vi "题目 3.vi"() -> ()   [LabVIEW 2017]
panel:
  out "数组":dbl[][](array[numeric])
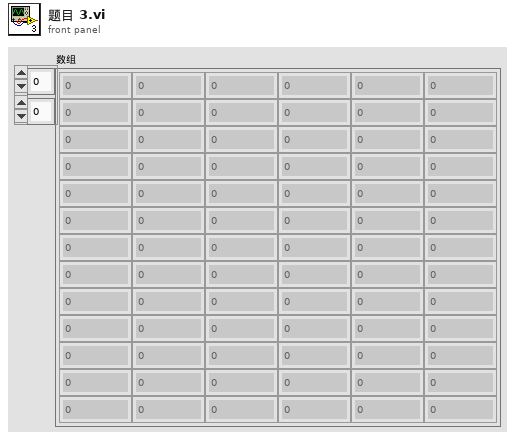
[diagram p1: front panel]
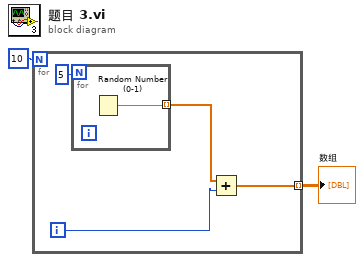
[diagram p0: block diagram]
diagram:
  n1 = for {
    N: 10 -> [_]
    tunnel: [w5] -> w1 mode=indexing
    i -> [w3]
    n2 = for {
      N: 5 -> [_]
      tunnel: [w7] -> w4 mode=indexing
      n3 = Random Number (0-1)() -> (number: 0 to 1=w7:dbl)
    }
    n4 = Add(x=w4, y=w3) -> (x+y=w5:dbl[])
  }
  "数组" <- w1
